vi "acel noise.vi"(9 "Pattern frequency (Hz)":dbl, 10 "Frecuencia de muestreo (Hz)":dbl, 11 "medidas":sgl[][](array[numeric])) -> (1 "Continuar?":bool, 2 "Report":string, 3 "medidas out":sgl[][](array[numeric]))   [LabVIEW 2015]
uses:
  <vilib>/Analysis/5stat.llb/RMS (DBL).vi
  <vilib>/measure/madcrms.llb/Basic Averaged DC-RMS for 1 Chan.vi
  <vilib>/measure/NI_MAPro.lvlib
  <vilib>/Analysis/NI_AALPro.lvlib
  <vilib>/Analysis/NI_AALBase.lvlib
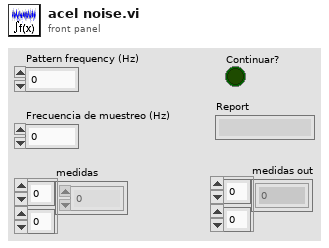
[diagram p1: front panel]
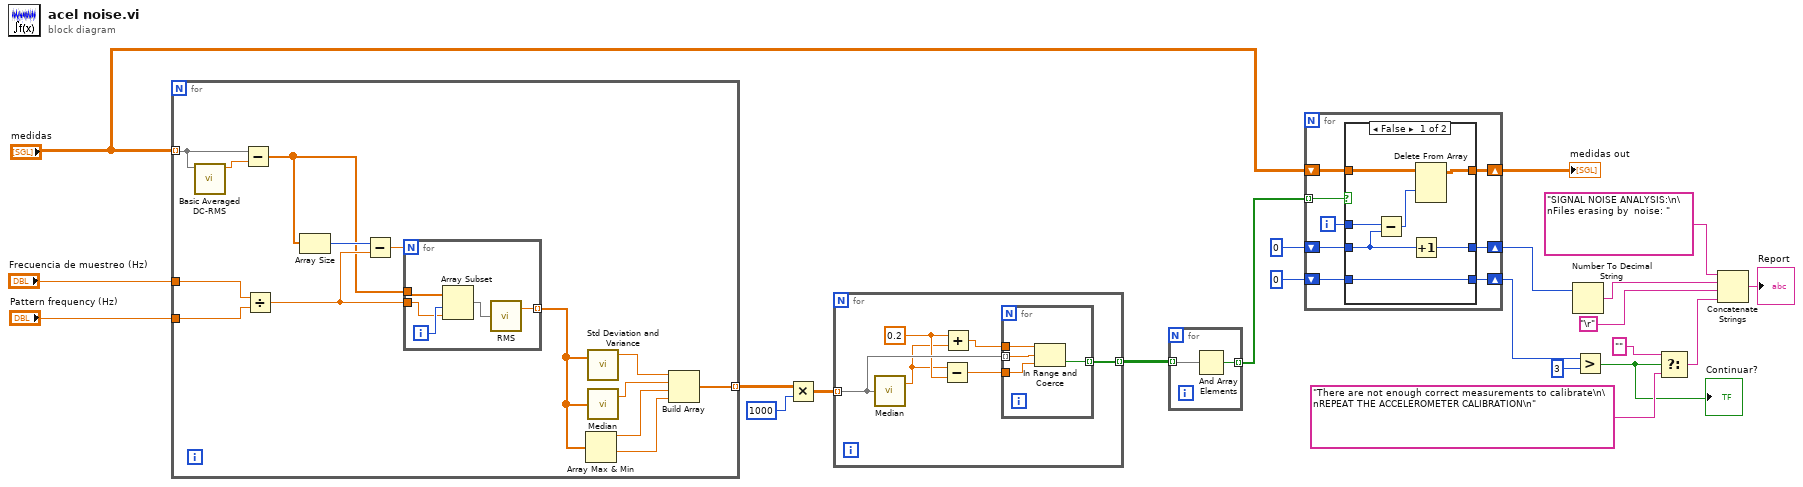
[diagram p0: block diagram]
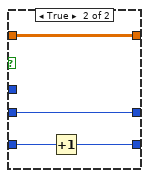
[diagram p2: hidden frame]
diagram:
  n1 = for {
    tunnel: "medidas" -> [w23] mode=indexing
    tunnel: [w29] -> w17 mode=indexing
    tunnel: "Frecuencia de muestreo (Hz)" -> [w24]
    tunnel: "Pattern frequency (Hz)" -> [w25]
    n2 = call-poly <vilib>:"Basic Averaged DC-RMS.vi"("signal in"=w23) -> ("DC value"=w36:dbl)  [unwired: 7 in, 3 out]
    n3 = Subtract(x=w23, y=w36) -> (x-y=w26:dbl[])
    n4 = Divide(x=w24, y=w25) -> (x/y=w33:dbl)
    n5 = Array Size(array=w26) -> (size(s)=w34:i32)
    n6 = Subtract(x=w34, y=w33) -> (x-y=w35:dbl)
    n7 = for {
      N: w35 -> [_]
      tunnel: w33 -> [w38]
      tunnel: [w41] -> w27 mode=indexing
      tunnel: w26 -> [w40]
      i -> [w39]
      n8 = Array Subset(array=w40, index=w39, length=w38) -> (w37:dbl[])
      n9 = call-poly <vilib>:"RMS.vi"("X"=w37) -> ("rms value"=w41:dbl)  [unwired: 1 out]
    }
    n10 = Array Max & Min(array=w27) -> (max value=w31:dbl, min value=w30:dbl)  [unwired: 2 out]
    n11 = call <vilib>:"Std Deviation and Variance.vi"("X"=w27) -> ("mean"=w28:dbl)  [unwired: 1 in, 2 out]
    n12 = call <vilib>:"Median.vi"("X"=w27) -> ("median"=w32:dbl)  [unwired: 1 out]
    n13 = Build Array(w28, w32, w31, w30) -> (w29:dbl[])
  }
  n14 = Multiply(x=w17, y=1000 ("median")) -> (x*y=w19:dbl[][])
  n15 = for {
    tunnel: w19 -> [w47] mode=indexing
    tunnel: [w42] -> w18 mode=indexing
    w45 = 0.2 ("x")
    n16 = call <vilib>:"Median.vi"("X"=w47) -> ("median"=w43:dbl)  [unwired: 1 out]
    n17 = Subtract(x=w43, y=w45) -> (x-y=w44:dbl)
    n18 = Add(x=w45, y=w43) -> (x+y=w46:dbl)
    n19 = for {
      tunnel: w47 -> [w51] mode=indexing
      tunnel: w46 -> [w50]
      tunnel: w44 -> [w49]
      tunnel: [w48] -> w42 mode=indexing
      n20 = In Range and Coerce(upper limit=w50, x=w51, lower limit=w49) -> (In Range?=w48:bool)  [unwired: 1 out]
    }
  }
  n21 = for {
    tunnel: w18 -> [w53] mode=indexing
    tunnel: [w52] -> w3 mode=indexing
    n22 = And Array Elements(Boolean array=w53) -> (logical AND=w52:bool)
  }
  n23 = for {
    shift-right: [w60] -> w1
    shift-left: "medidas" -> [w61]
    tunnel: w3 -> [w59] mode=indexing
    shift-right: [w56] -> w15
    shift-left: 0 ("index of element") -> [w57]
    shift-right: [w54] -> w10
    shift-left: 0 ("index of element") -> [w55]
    i -> [w58]
    n24 = case shown="False" w59 {
      tunnel: w61 -> [w68 w72]
      tunnel: [w67 w72] -> w60
      tunnel: w58 -> [w66 _]
      tunnel: w57 -> [w65 w71]
      tunnel: [w64 w71] -> w56
      tunnel: w55 -> [w63 w70]
      tunnel: [w63 w69] -> w54
      frame False {
        n25 = Subtract(x=w66, y=w65) -> (x-y=w62:i32)
        n26 = Increment(x=w65) -> (x+1=w64:i32)
        n27 = Delete From Array(array=w68, index (row)=w62) -> (array with subset deleted=w67:sgl[][])  [unwired: 2 in, 1 out]
      }
      frame True {
        n28 = Increment(x=w70) -> (x+1=w69:i32)
      }
    }
  }
  "medidas out" <- w1
  n29 = Number To Decimal String(number=w15) -> (decimal integer string=w13:string)  [unwired: 1 in]
  n30 = Greater?(x=w10, y=3) -> (0:w5:bool)
  "Continuar?" <- w5
  n31 = Select(t="", s=w5, f="There are not enough correct measurements to calibrate\n\nREPEAT THE ACCELEROMETER CALIBRATION\n") -> (s? t:f=w6:string)
  n32 = Concatenate Strings("SIGNAL NOISE ANALYSIS:\n\nFiles erasing by  noise: ", w13, "\r", w6) -> (→"Report":string)
